vi "Simple Timer.vi"(10 "Target [s]":dbl=5.0, 11 "Timing?":bool) -> (2 "Timer Value":dbl, 3 "Target Reached":bool)   [LabVIEW 2019]
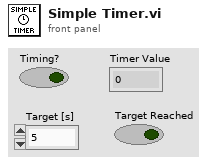
[diagram p1: front panel]
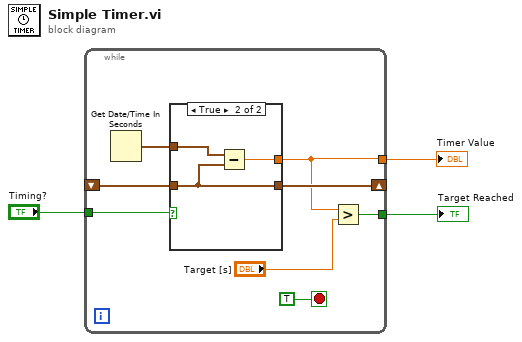
[diagram p0: block diagram]
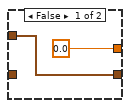
[diagram p2: hidden frame]
diagram:
  n1 = while {
    tunnel: "Timing?" -> [w10]
    shift-right: [w9] -> _
    shift-left: _ -> [w7]
    tunnel: [w6] -> w2
    tunnel: [w4] -> w3
    stop <- TRUE stop-if-true
    n2 = Get Date/Time In Seconds() -> (seconds since 1Jan1904=w8:timestamp)
    n3 = case shown="True" w10 {
      tunnel: [w13 w15] -> w9
      tunnel: w8 -> [w13 w16]
      tunnel: w7 -> [_ w15]
      tunnel: [0.0 w14] -> w6
      frame False {
      }
      frame True {
        n4 = Subtract(x=w16, y=w15) -> (x-y=w14:dbl)
      }
    }
    n5 = Greater?(x=w6, y="Target [s]") -> (0:w4:bool)
  }
  "Target Reached" <- w3
  "Timer Value" <- w2
